vi "Escape and Enclose String.vi"(7 "Force Enclose? (F)":bool, 11 "String":string) -> (3 "JSON String":string)   [LabVIEW 2018, in "JSON.lvlib"]
uses:
  JSON.lvlib
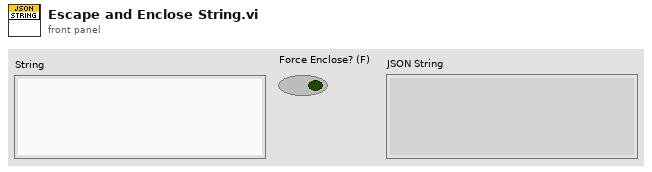
[diagram p1: front panel]
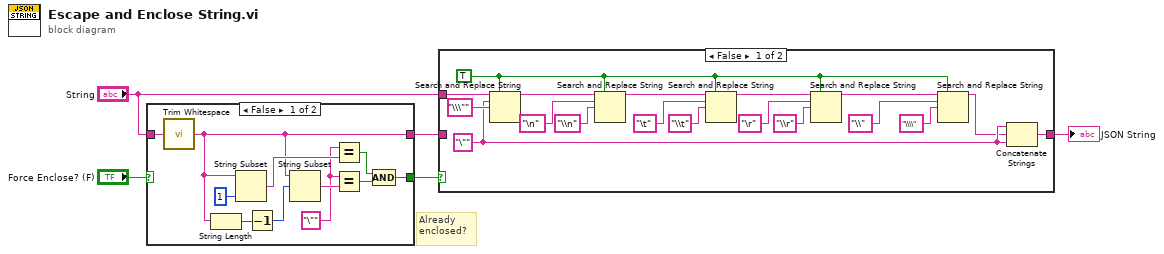
[diagram p0: block diagram]
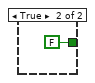
[diagram p2: hidden frame]
diagram:
  # "Already enclosed?"
  n1 = case shown="False" "Force Enclose? (F)" {
    tunnel: "String" -> [w8 _]
    tunnel: [w7 FALSE] -> w4
    tunnel: [w6 _] -> w2
    frame False {
      w11 = "\"" ("x")
      n2 = call <vilib>:"Trim Whitespace.vi"("string"=w8) -> ("trimmed string"=w6:string)  [unwired: 1 in]
      n3 = String Length(string=w6) -> (length=w15:i32)
      n4 = String Subset(string=w6, length (rest)=1 ("length (rest)")) -> (substring=w13:string)  [unwired: 1 in]
      n5 = Decrement(x=w15) -> (x-1=w14:i32)
      n6 = String Subset(string=w6, offset (0)=w14) -> (substring=w12:string)  [unwired: 1 in]
      n7 = Equal?(x=w11, y=w13) -> (x = y?=w10:bool)
      n8 = Equal?(x=w11, y=w12) -> (x = y?=w9:bool)
      n9 = Compound Arithmetic op=AND(w10, w9) -> (w7:bool)
    }
    frame True {
    }
  }
  n10 = case shown="False" w4 {
    tunnel: w2 -> [_ w36]
    tunnel: "String" -> [w35 _]
    tunnel: [w33 w36] -> w3
    frame False {
      w19 = TRUE ("replace all? (F)")
      w32 = "\"" ("search string")
      n11 = Search and Replace String(replace all?=w19, input string=w35, search string=w32, replace string="\\\"" ("replace string (\"\")")) -> (result string=w30:string)  [unwired: 4 in, 3 out]
      n12 = Search and Replace String(replace all?=w19, input string=w30, search string="\n" ("replace string (\"\")"), replace string="\\n" ("replace string (\"\")")) -> (result string=w26:string)  [unwired: 4 in, 3 out]
      n13 = Search and Replace String(replace all?=w19, input string=w26, search string="\t" ("replace string (\"\")"), replace string="\\t" ("replace string (\"\")")) -> (result string=w23:string)  [unwired: 4 in, 3 out]
      n14 = Search and Replace String(replace all?=w19, input string=w23, search string="\r" ("replace string (\"\")"), replace string="\\r" ("replace string (\"\")")) -> (result string=w20:string)  [unwired: 4 in, 3 out]
      n15 = Search and Replace String(replace all?=w19, input string=w20, search string="\\" ("replace string (\"\")"), replace string="\\\\" ("replace string (\"\")")) -> (result string=w18:string)  [unwired: 4 in, 3 out]
      n16 = Concatenate Strings(w32, w18, w32) -> (w33:string)
    }
    frame True {
    }
  }
  "JSON String" <- w3
